vi "growing_gauss.vi"() -> ()   [LabVIEW 2015]
panel:
  out "z_values":dbl[](array[numeric])
  out "y_values":dbl[](array[numeric])
  out "x_values":dbl[](array[numeric])
  out "z_i":dbl
  out "y_i":dbl
  out "x_i":dbl
  out "len(z)":i32
  out "len(y)":i32
  out "len(x)":i32
  out "Intensity Graph":dbl[][](graph)
  in  "sigma":sgl
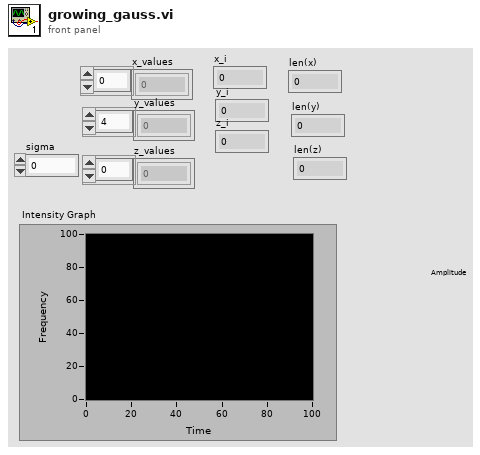
[diagram p1: front panel]
types:
  T1 = enum16{"open", "replace", "create", "open or create", "replace or create", "replace or create with confirmation"}
  T2 = enum16{"big-endian, network order", "native, host order", "little-endian"}
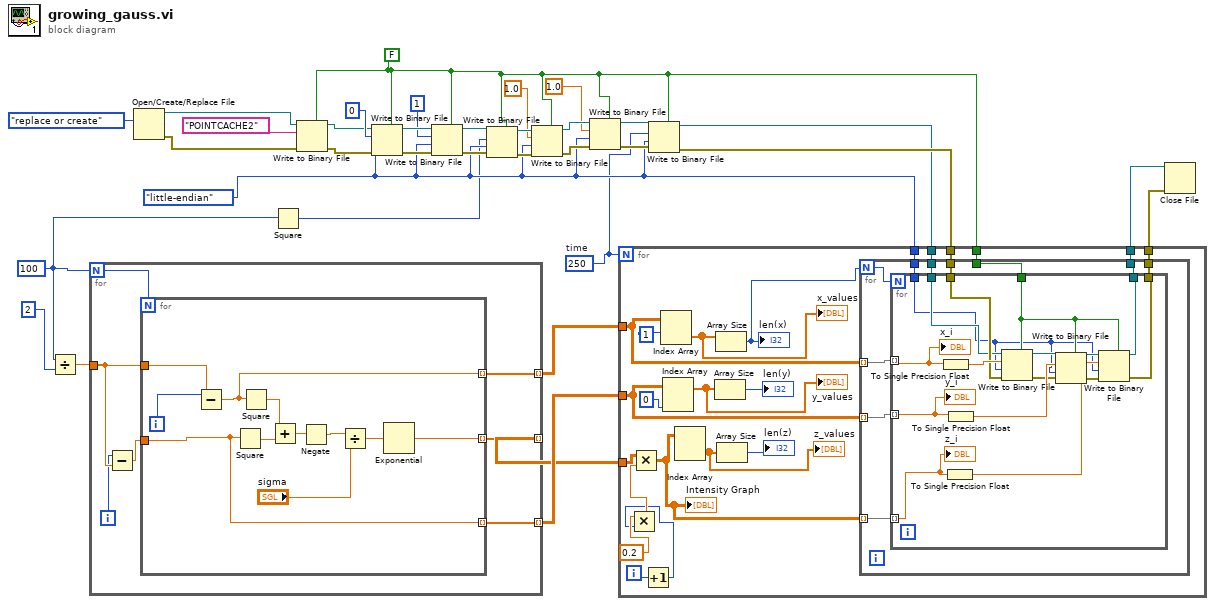
[diagram p0: block diagram]
diagram:
  w6 = FALSE ("prepend array or string size? (T)")
  w7 = T2."little-endian" ("byte order (0:big-endian, network order)")
  w3 = 250  # time
  w2 = 100
  n1 = Divide(x=w2, y=2) -> (x/y=w33:dbl)
  n2 = for {
    N: w2 -> [w41]
    tunnel: w33 -> [w40]
    tunnel: [w37] -> w10 mode=indexing
    tunnel: [w36] -> w12 mode=indexing
    tunnel: [w35] -> w11 mode=indexing
    i -> [w39]
    n3 = Subtract(x=w39, y=w40) -> (x-y=w38:dbl)
    n4 = for {
      N: w41 -> [_]
      tunnel: w40 -> [w52]
      tunnel: w38 -> [w42]
      tunnel: [w44] -> w37 mode=indexing
      tunnel: [w43] -> w36 mode=indexing
      tunnel: [w42] -> w35 mode=indexing
      i -> [w51]
      n5 = Subtract(x=w51, y=w52) -> (x-y=w43:dbl)
      n6 = Square(x=w42) -> (x^2=w49:dbl)
      n7 = Square(x=w43) -> (x^2=w50:dbl)
      n8 = Add(x=w50, y=w49) -> (x+y=w48:dbl)
      n9 = Negate(x=w48) -> (-x=w47:dbl)
      n10 = Divide(x=w47, y="sigma") -> (x/y=w45:dbl)
      n11 = Exponential(1:w45) -> (0:w44:dbl)
    }
  }
  n12 = Open/Create/Replace File(operation (0:open)=T1."replace or create") -> (refnum out=w13:refnum<file>, error out=w14:errorcluster)  [unwired: 5 in, 1 out]
  n13 = Square(x=w2) -> (x^2=w1:i32)
  n14 = Write to Binary File(file (use dialog)=w13, data="POINTCACHE2", error in=w14, 5:w6) -> (refnum out=w16:refnum<file>, error out=w15:errorcluster)  [unwired: 2 in, 1 out]
  n15 = Write to Binary File(file (use dialog)=w16, data=i8 0, error in=w15, 5:w6, 9:w7) -> (refnum out=w22:refnum<file>, error out=w23:errorcluster)  [unwired: 1 in, 1 out]
  n16 = Write to Binary File(file (use dialog)=w22, data=1, error in=w23, 5:w6, 9:w7) -> (refnum out=w20:refnum<file>, error out=w19:errorcluster)  [unwired: 1 in, 1 out]
  n17 = Write to Binary File(file (use dialog)=w20, data=w1, error in=w19, 5:w6, 9:w7) -> (refnum out=w31:refnum<file>, error out=w26:errorcluster)  [unwired: 1 in, 1 out]
  n18 = Write to Binary File(file (use dialog)=w31, data=sgl 1.0, error in=w26, 5:w6, 9:w7) -> (refnum out=w30:refnum<file>, error out=w25:errorcluster)  [unwired: 1 in, 1 out]
  n19 = Write to Binary File(file (use dialog)=w30, data=sgl 1.0, error in=w25, 5:w6, 9:w7) -> (refnum out=w27:refnum<file>, error out=w24:errorcluster)  [unwired: 1 in, 1 out]
  n20 = Write to Binary File(file (use dialog)=w27, data=w3, error in=w24, 5:w6, 9:w7) -> (refnum out=w8:refnum<file>, error out=w9:errorcluster)  [unwired: 1 in, 1 out]
  n21 = for {
    N: w3 -> [_]
    tunnel: w12 -> [w62]
    tunnel: w11 -> [w63]
    tunnel: w10 -> [w73]
    tunnel: w9 -> [w60]
    tunnel: w8 -> [w59]
    tunnel: w7 -> [w58]
    tunnel: w6 -> [w61]
    tunnel: [w57] -> w5
    tunnel: [w56] -> w4
    i -> [w74]
    n22 = Increment(x=w74) -> (x+1=w53:i32)
    n23 = Multiply(x=0.2, y=w53) -> (x*y=w55:dbl)
    n24 = Multiply(x=w73, y=w55) -> (x*y=w64:dbl[][])
    "Intensity Graph" <- w64
    n25 = Index Array(array=w62, index (row)=1) -> (element=w69:dbl[])  [unwired: 1 in]
    "x_values" <- w69
    n26 = Index Array(array=w63, index (col)=0 ("index (row)")) -> (element=w68:dbl[])  [unwired: 1 in]
    "y_values" <- w68
    n27 = Index Array(array=w64) -> (element=w67:dbl[])  [unwired: 2 in]
    "z_values" <- w67
    n28 = Array Size(array=w68) -> (size(s)=→"len(y)":i32)
    n29 = Array Size(array=w69) -> (size(s)=w65:i32)
    "len(x)" <- w65
    n30 = Array Size(array=w67) -> (size(s)=→"len(z)":i32)
    n31 = for {
      N: w65 -> [w84]
      tunnel: w64 -> [w83] mode=indexing
      tunnel: w63 -> [w82] mode=indexing
      tunnel: w62 -> [w81] mode=indexing
      tunnel: w61 -> [w80]
      tunnel: w60 -> [w79]
      tunnel: w59 -> [w78]
      tunnel: w58 -> [w77]
      tunnel: [w76] -> w57
      tunnel: [w75] -> w56
      n32 = for {
        N: w84 -> [_]
        tunnel: w81 -> [w99] mode=indexing
        tunnel: w82 -> [w100] mode=indexing
        tunnel: [w93] -> w76
        tunnel: [w92] -> w75
        tunnel: w83 -> [w94] mode=indexing
        tunnel: w80 -> [w88]
        tunnel: w79 -> [w87]
        tunnel: w78 -> [w86]
        tunnel: w77 -> [w85]
        n33 = To Single Precision Float(number=w99) -> (single precision float=w98:sgl)
        n34 = To Single Precision Float(number=w94) -> (single precision float=w89:sgl)
        n35 = To Single Precision Float(number=w100) -> (single precision float=w97:sgl)
        n36 = Write to Binary File(file (use dialog)=w86, data=w98, error in=w87, 5:w88, 9:w85) -> (refnum out=w95:refnum<file>, error out=w96:errorcluster)  [unwired: 1 in, 1 out]
        n37 = Write to Binary File(file (use dialog)=w95, data=w97, error in=w96, 5:w88, 9:w85) -> (refnum out=w90:refnum<file>, error out=w91:errorcluster)  [unwired: 1 in, 1 out]
        n38 = Write to Binary File(file (use dialog)=w90, data=w89, error in=w91, 5:w88, 9:w85) -> (refnum out=w93:refnum<file>, error out=w92:errorcluster)  [unwired: 1 in, 1 out]
        "x_i" <- w99
        "y_i" <- w100
        "z_i" <- w94
      }
    }
  }
  n39 = Close File(refnum=w5, error in=w4) -> ()  [unwired: 2 out]
